vi "16TVTIMonitor.vi"() -> ()   [LabVIEW 2016]
uses:
  Utility/Monitor Communication/S16/VTI-cluster.ctl
  Utility/Monitor Communication/S16/VTI-control.ctl
  Instrument_Setup.vi
  Global/Global Variables/Data_Display_global.vi
panel:
  out "VTI":T1={"Temperatur (K)"=0.0, "Setpoint (K)"=0.0, "Rate (K/min)"=3.4572, "Heater (%)"=0.0, "NV (%)"=0.0, "Heater Manual"=FALSE, "NV Manual"=FALSE, "Go to Set"=FALSE, "Pressure"=0.0, "Heater SP"=0.0, "Valid?"=FALSE, "Set Heater SP"=FALSE, "Set NV SP"=FALSE, "Heater (%) Display"=3.4572, "NV (%) Display"=3.4572, "NV Setpoint"=0.0, "Change Heater Status"=FALSE, "Change NV Status"=FALSE, "Sample 3"=0.0, "Sample 2"=0.0, "Sweep-State"=FALSE, "Set Auto PID"=FALSE, "Auto PID"=FALSE, "Stopp"=FALSE, "Setpoint-Sweep"=0.0} {"NV (%) Display" format="%4_5f"; "Heater (%) Display" format="%4_5f"; "Pressure" format="%#4_5f"; "NV (%)" scale=0.0..100.0; "Heater (%)" scale=0.0..100.0; "Rate (K/min)" format="%#4_5f"; "Setpoint (K)" format="%6_5f"}
  in  "local error":errorcluster
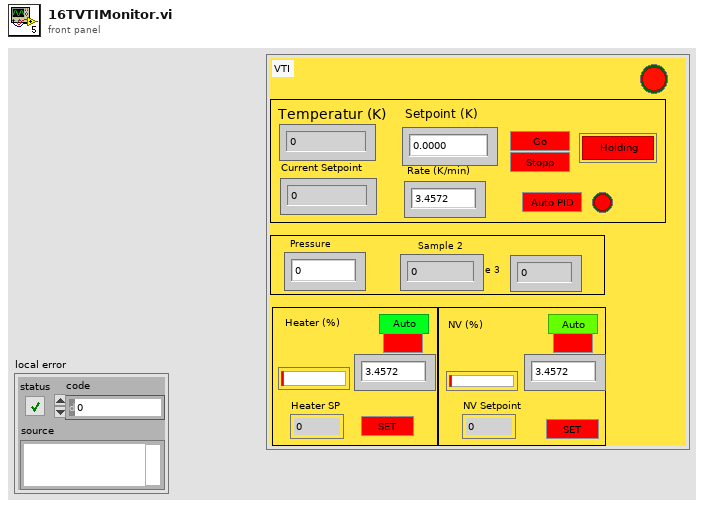
[diagram p1: front panel]
types:
  T1 = typedef "VTI-cluster.ctl" = cluster{"Temperatur (K)":dbl, "Setpoint (K)":dbl, "Rate (K/min)":dbl, "Heater (%)":dbl, "NV (%)":dbl, "Heater Manual":bool, "NV Manual":bool, "Go to Set":bool, "Pressure":dbl, "Heater SP":dbl, "Valid?":bool, "Set Heater SP":bool, "Set NV SP":bool, "Heater (%) Display":dbl, "NV (%) Display":dbl, "NV Setpoint":dbl, "Change Heater Status":bool, "Change NV Status":bool, "Sample 3":dbl, "Sample 2":dbl, "Sweep-State":bool, "Set Auto PID":bool, "Auto PID":bool, "Stopp":bool, "Setpoint-Sweep":dbl}
  T2 = typedef "VTI-control.ctl" = cluster{"Set VTI SP":bool, "Change NV Status":bool, "Set NV Setpoint":bool, "Change Heater Status":bool, "Set Heater Setpoint":bool, "Setpoint (K)":dbl, "Rate (K/min)":dbl, "Setpoint Heater":dbl, "Setpoint NV":dbl, "Change Auto PID":bool, "Stop Sweep":bool}
  T3 = typedef "ITCVersion.ctl" = enum16{"ITC502", "ITC503", "ITC601"}
  T4 = cluster{"Version":T3, "ControlTITC":i8, "ControlTCh":i8, "SampleTITC":i8, "SampleTCh":i8, "Instrument address":cluster{"Com Port":i32, "ISOBUS Address":i32, "GPIB Address":i16, "Communication":enum16{"RS232", "ISOBUS", "GPIB", "Gateway"}}}
  T5 = cluster{"Com Port":i32, "ISOBUS Address":i32, "GPIB Address":i16, "Communication":enum16{"RS232", "ISOBUS", "GPIB", "Gateway"}}
  T6 = enum32{"Bad", "Idle", "Run top level", "Running"}
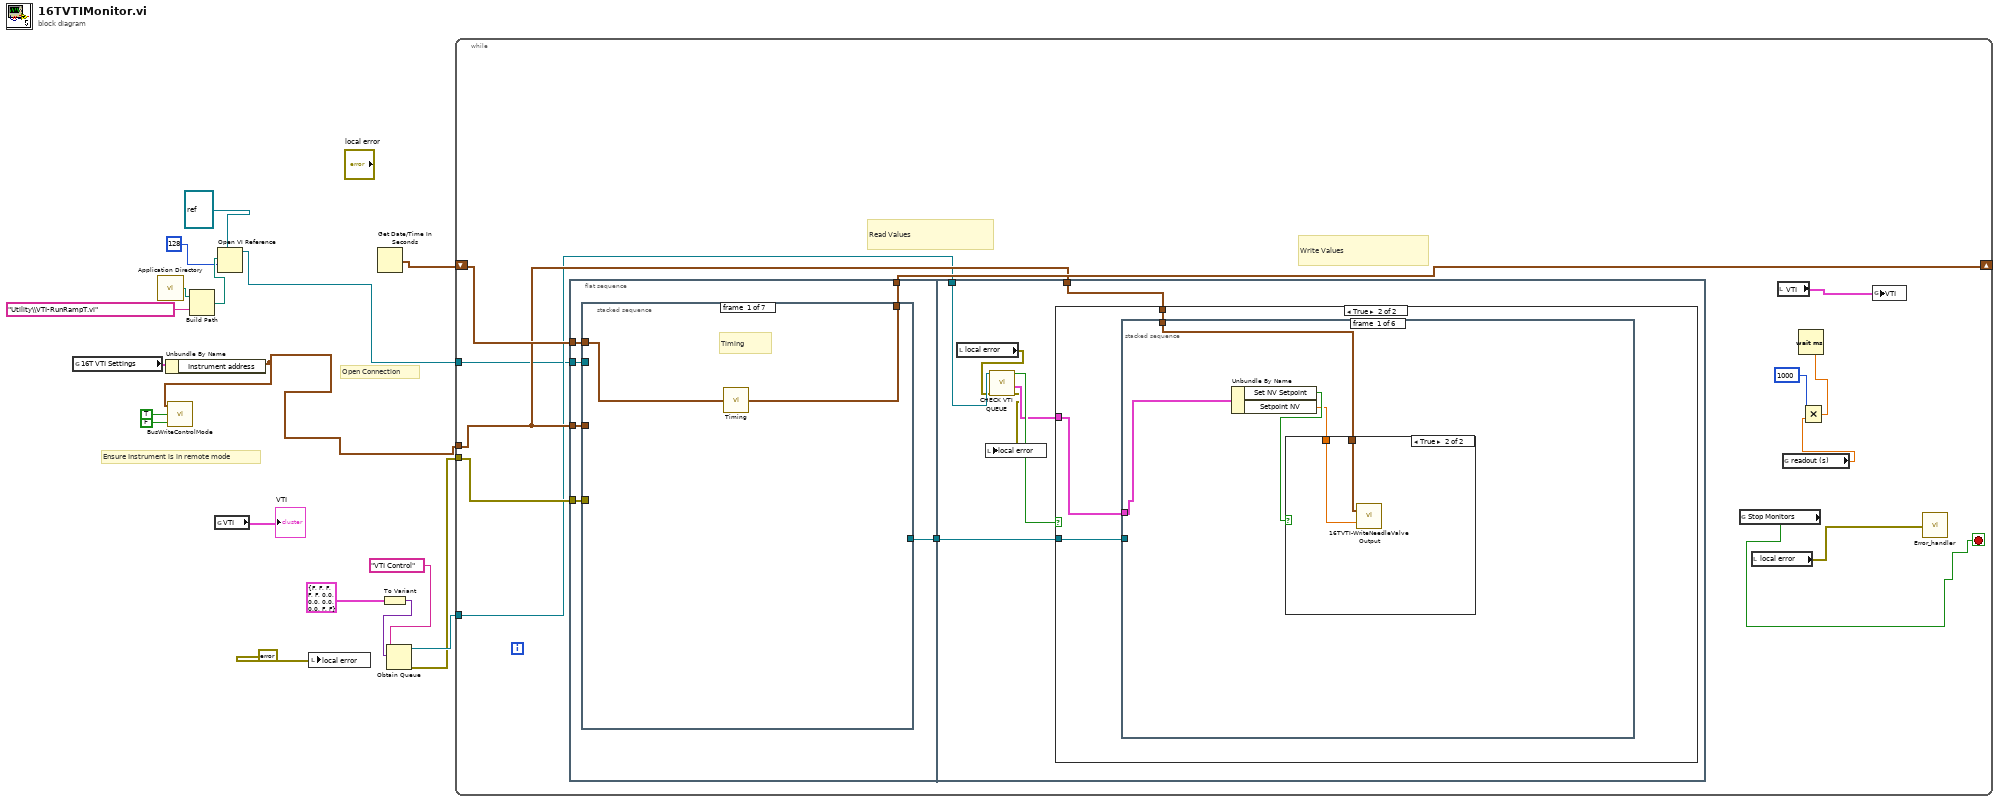
[diagram p0: block diagram]
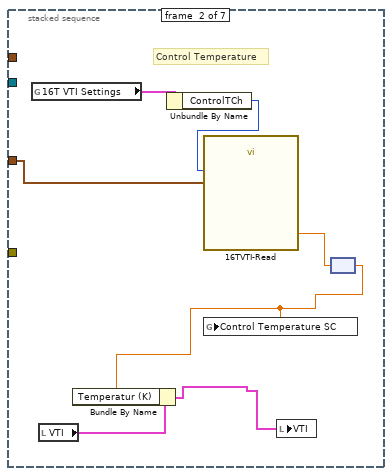
[diagram p2: hidden frame]
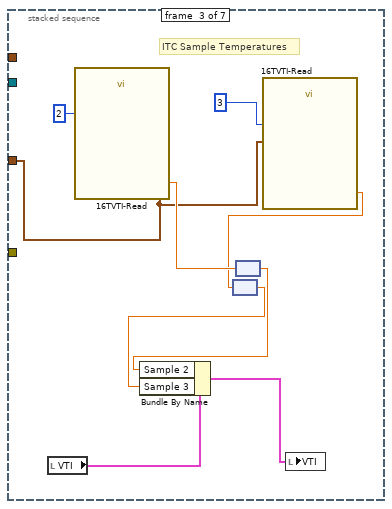
[diagram p3: hidden frame]
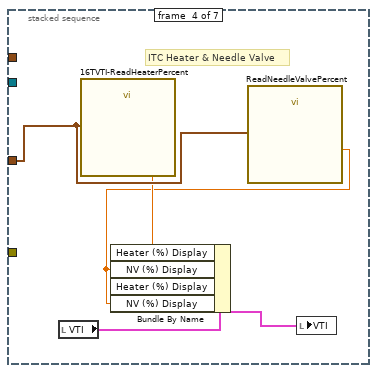
[diagram p4: hidden frame]
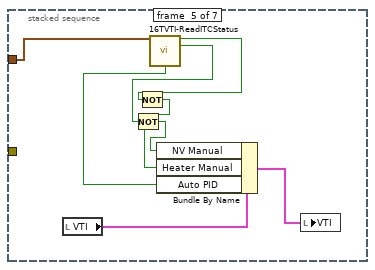
[diagram p5: hidden frame]
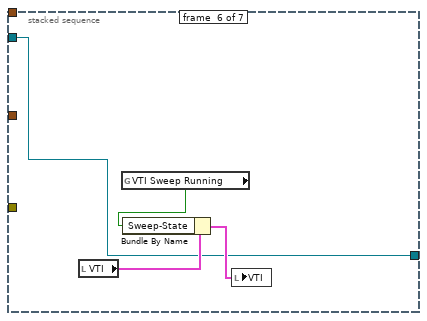
[diagram p6: hidden frame]
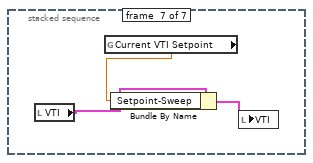
[diagram p7: hidden frame]
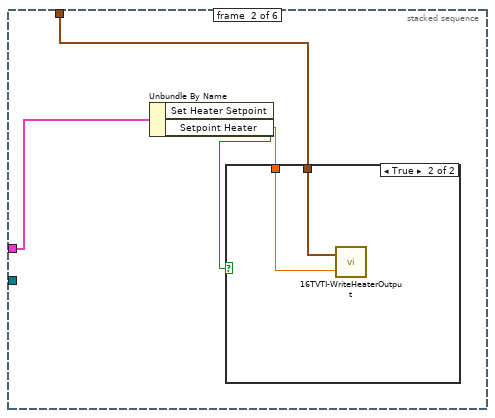
[diagram p10: hidden frame]
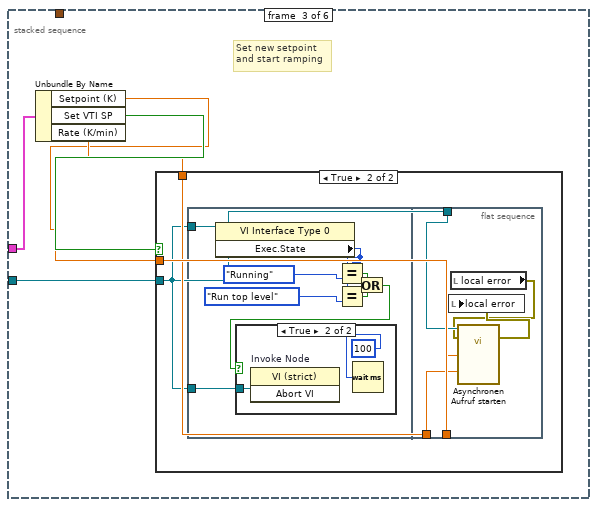
[diagram p12: hidden frame]
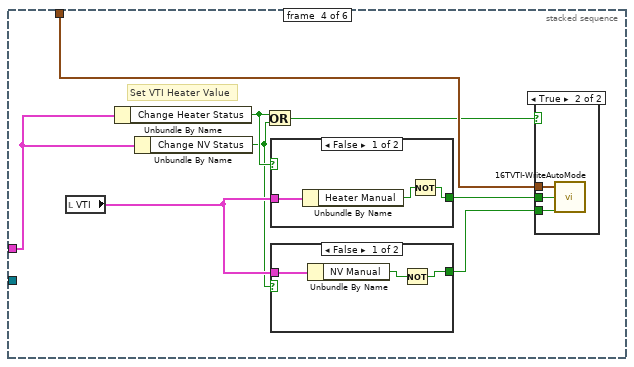
[diagram p15: hidden frame]
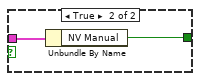
[diagram p17: hidden frame]
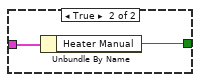
[diagram p18: hidden frame]
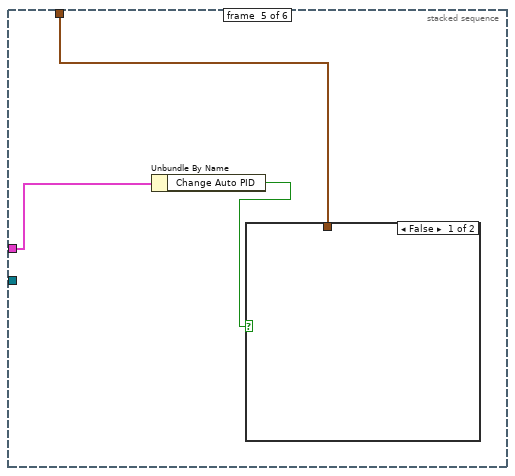
[diagram p19: hidden frame]
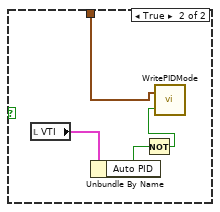
[diagram p20: hidden frame]
diagram:
  # "Ensure Instrument is in remote mode"
  # "Open Connection"
  n1 = global read "Instrument_Setup.vi" "16T VTI Settings"() -> (w4:T4)
  n2 = call <vilib>:"Application Directory.vi"() -> ("Application Directory"=w10:path)
  n3 = Unbundle By Name(w4) -> ("Instrument address"=w1:T5)
  n4 = call "BusWriteControlMode.vi"("Locked"=FALSE, "Remote"=TRUE, "Address"=w1) -> ()  [unwired: 1 out]
  n5 = Build Path(base path=w10, name or relative path="Utility\\VTI-RunRampT.vi") -> (appended path=w8:path)
  n6 = global read "Data_Display_global.vi" "VTI"() -> (→"VTI":T1)
  n7 = Open VI Reference(type specifier VI Refnum (for type only)=refnum<vi> refnum ("vi reference"), vi path=w8, options=128) -> (vi reference=w5:refnum<vi>)  [unwired: 3 in, 1 out]
  n8 = local write "local error"(errorcluster {"status"=FALSE, "code"=0, "source"=""} ("error constant")) -> ()
  n9 = Get Date/Time In Seconds() -> (seconds since 1Jan1904=w18:timestamp)
  n10 = To Variant(anything=T2 {"Set VTI SP"=FALSE, "Change NV Status"=FALSE, "Set NV Setpoint"=FALSE, "Change Heater Status"=FALSE, "Set Heater Setpoint"=FALSE, "Setpoint (K)"=0.0, "Rate (K/min)"=0.0, "Setpoint Heater"=0.0, "Setpoint NV"=0.0, "Change Auto PID"=FALSE, "Stop Sweep"=FALSE} ("VTI Control")) -> (Variant=w17:variant)
  n11 = Obtain Queue(name (unnamed)="VTI Control", element data type=w17) -> (queue out=w15:refnum<queue>, error out=w14:errorcluster)  [unwired: 3 in, 1 out]
  n12 = while {
    tunnel: w1 -> [w25]
    tunnel: w14 -> [w31]
    shift-right: [w26] -> _
    shift-left: w18 -> [w27]
    tunnel: w15 -> [w23]
    tunnel: w5 -> [w20]
    stop <- w21 stop-if-true
    # "Write Values"
    # "Read Values"
    n13 = flat-sequence {
      tunnel: w31 -> [w37]
      tunnel: w25 -> [w36]
      tunnel: w27 -> [w35]
      tunnel: [w34] -> w26
      tunnel: w20 -> [w33]
      tunnel: [w32] -> w19
      tunnel: w25 -> [w82]
      tunnel: w23 -> [w81]
      tunnel: w19 -> [w76]
      frame #0 {
        n14 = stacked-sequence {
          tunnel: w36 -> [_ w46 w50 w60 w64 _ _]
          tunnel: w37 -> [_ _ _ _ _ _ _]
          tunnel: w35 -> [w39 _ _ _ _ _ _]
          tunnel: [w38 _ _ _ _ _ _] -> w34
          tunnel: w33 -> [_ _ _ _ _ w70 _]
          tunnel: [_ _ _ _ _ w70 _] -> w32
          frame #0 {
            # "Timing"
            n15 = call "Timing.vi"("start time (s)"=w39) -> ("last reading (s)"=w38:timestamp)
          }
          frame #1 {
            # "Control Temperature"
            n16 = global read "Instrument_Setup.vi" "16T VTI Settings"() -> (w41:T4)
            n17 = local read "VTI"() -> (w45:T1)
            n18 = Unbundle By Name(w41) -> ("ControlTCh"=w40:i8)
            n19 = call "16TVTI-Read.vi"("Channel"=w40, "IO Info"=w46) -> ("Temperature"=w43:dbl[unit])  [unwired: 3 in, 2 out]
            n20 = node(w43) -> (w42:dbl)
            n21 = Bundle By Name(cluster=w45, "Temperatur (K)"=w42) -> (w44:T1)
            n22 = global write "Data_Display_global.vi" "Control Temperature SC"(w42) -> ()
            n23 = local write "VTI"(w44) -> ()
          }
          frame #2 {
            # "ITC Sample Temperatures"
            n24 = local read "VTI"() -> (w53:T1)
            n25 = call "16TVTI-Read.vi"("Channel"=i16 2, "IO Info"=w50) -> ("Temperature"=w54:dbl[unit])  [unwired: 3 in, 2 out]
            n26 = node(w54) -> (w48:dbl)
            n27 = call "16TVTI-Read.vi"("Channel"=i16 3, "IO Info"=w50) -> ("Temperature"=w49:dbl[unit])  [unwired: 3 in, 2 out]
            n28 = node(w49) -> (w47:dbl)
            n29 = Bundle By Name(cluster=w53, "Sample 2"=w48, "Sample 3"=w47) -> (w52:T1)
            n30 = local write "VTI"(w52) -> ()
          }
          frame #3 {
            # "ITC Heater & Needle Valve"
            n31 = local read "VTI"() -> (w58:T1)
            n32 = call "16TVTI-ReadHeaterPercent.vi"("ITC IO Info"=w60) -> ("Actual heater  %"=w57:dbl)  [unwired: 1 in, 1 out]
            n33 = call "ReadNeedleValvePercent.vi"("IO Info"=w60) -> ("Actual Needle Valve  %"=w56:dbl)  [unwired: 1 in, 1 out]
            n34 = Bundle By Name(cluster=w58, "Heater (%) Display"=w57, "NV (%) Display"=w56, "Heater (%) Display"=w57, "NV (%) Display"=w56) -> (w59:T1)
            n35 = local write "VTI"(w59) -> ()
          }
          frame #4 {
            n36 = local read "VTI"() -> (w68:T1)
            n37 = call "16TVTI-ReadITCStatus.vi"("ITC IO Info"=w64) -> ("Auto heat"=w66:bool, "Auto Needle Valve"=w65:bool, "Auto PID"=w61:bool)  [unwired: 4 in, 8 out]
            n38 = Not(x=w65) -> (.not. x?=w63:bool)
            n39 = Not(x=w66) -> (.not. x?=w62:bool)
            n40 = Bundle By Name(cluster=w68, "NV Manual"=w63, "Heater Manual"=w62, "Auto PID"=w61) -> (w67:T1)
            n41 = local write "VTI"(w67) -> ()
          }
          frame #5 {
            n42 = local read "VTI"() -> (w72:T1)
            n43 = global read "Data_Display_global.vi" "VTI Sweep Running"() -> (w69:bool)
            n44 = Bundle By Name(cluster=w72, "Sweep-State"=w69) -> (w71:T1)
            n45 = local write "VTI"(w71) -> ()
          }
          frame #6 {
            n46 = local read "VTI"() -> (w75:T1)
            n47 = global read "Data_Display_global.vi" "Current VTI Setpoint"() -> (w73:dbl)
            n48 = Bundle By Name(cluster=w75, "Setpoint-Sweep"=w73) -> (w74:T1)
            n49 = local write "VTI"(w74) -> ()
          }
        }
      }
      frame #1 {
        n50 = local read "local error"() -> (w78:errorcluster)
        n51 = call "CHECK VTI QUEUE.vi"("error in (no error)"=w78, "queue"=w81) -> ("error out"=w77:errorcluster, "VTI Control"=w79:T2, "New Entries?"=w80:bool)  [unwired: 6 in]
        n52 = local write "local error"(w77) -> ()
        n53 = case shown="True" w80 {
          tunnel: w82 -> [_ w85]
          tunnel: w79 -> [_ w84]
          tunnel: w76 -> [_ w83]
          frame False {
          }
          frame True {
            n54 = stacked-sequence {
              tunnel: w85 -> [w87 w92 _ w124 w143 _]
              tunnel: w84 -> [w89 w93 w102 w128 w142 w153]
              tunnel: w83 -> [_ _ w98 _ _ w152]
              frame #0 {
                n55 = Unbundle By Name(w89) -> ("Set NV Setpoint"=w88:bool, "Setpoint NV"=w86:dbl)
                n56 = case shown="True" w88 {
                  tunnel: w87 -> [_ w91]
                  tunnel: w86 -> [_ w90]
                  frame False {
                  }
                  frame True {
                    n57 = call "16TVTI-WriteNeedleValveOutput.vi"("Needle Valve Output (%"=w90, "ITC IO Info"=w91) -> ()  [unwired: 1 in, 1 out]
                  }
                }
              }
              frame #1 {
                n58 = Unbundle By Name(w93) -> ("Set Heater Setpoint"=w95:bool, "Setpoint Heater"=w94:dbl)
                n59 = case shown="True" w95 {
                  tunnel: w92 -> [_ w97]
                  tunnel: w94 -> [_ w96]
                  frame False {
                  }
                  frame True {
                    n60 = call "16TVTI-WriteHeaterOutput.vi"("Heater Output (%)"=w96, "ITC IO Info"=w97) -> ()  [unwired: 1 in, 1 out]
                  }
                }
              }
              frame #2 {
                # "Set new setpoint \nand start ramping"
                n61 = Unbundle By Name(w102) -> ("Setpoint (K)"=w99:dbl, "Set VTI SP"=w101:bool, "Rate (K/min)"=w100:dbl)
                n62 = case shown="True" w101 {
                  tunnel: w99 -> [_ w105]
                  tunnel: w100 -> [_ w104]
                  tunnel: w98 -> [_ w103]
                  frame False {
                  }
                  frame True {
                    n63 = flat-sequence {
                      tunnel: w103 -> [w113]
                      tunnel: w103 -> [w106]
                      tunnel: w105 -> [w120]
                      tunnel: w104 -> [w119]
                      tunnel: w103 -> [w118]
                      frame #0 {
                        n64 = property class="VI Interface Type 0"(reference=w113) -> ("Exec.State"=w107:T6)  [unwired: 1 in, 2 out]
                        n65 = Equal?(x=w107, y=T6."Running" ("LS 370 Monitor 2")) -> (x = y?=w111:bool)
                        n66 = Equal?(x=w107, y=T6."Run top level" ("LS 370 Monitor 2")) -> (x = y?=w112:bool)
                        n67 = Or(x=w111, y=w112) -> (x .or. y?=w110:bool)
                        n68 = case shown="True" w110 {
                          tunnel: w106 -> [_ w115]
                          frame False {
                          }
                          frame True {
                            n69 = invoke on="Invoke Node" class="VI (strict)" method="Abort VI"(reference=w115) -> ()  [unwired: 2 in, 3 out]
                            n70 = Wait (ms)(milliseconds to wait=100) -> ()  [unwired: 1 out]
                          }
                        }
                      }
                      frame #1 {
                        n71 = local read "local error"() -> (w116:errorcluster)
                        n72 = call-by-ref "Asynchronen Aufruf starten"(reference=w118, error in=w116, "Rate (K/min)"=w119, "Final T (K)"=w120) -> (error out=w117:errorcluster)  [unwired: 2 out]
                        n73 = local write "local error"(w117) -> ()
                      }
                    }
                  }
                }
              }
              frame #3 {
                # "Set VTI Heater Value"
                n74 = local read "VTI"() -> (w127:T1)
                n75 = Unbundle By Name(w128) -> ("Change Heater Status"=w123:bool)
                n76 = Unbundle By Name(w128) -> ("Change NV Status"=w121:bool)
                n77 = Or(x=w123, y=w121) -> (x .or. y?=w122:bool)
                n78 = case shown="False" w123 {
                  tunnel: w127 -> [w139 w141]
                  tunnel: [w137 w140] -> w125
                  frame False {
                    n79 = Unbundle By Name(w139) -> ("Heater Manual"=w138:bool)
                    n80 = Not(x=w138) -> (.not. x?=w137:bool)
                  }
                  frame True {
                    n81 = Unbundle By Name(w141) -> ("Heater Manual"=w140:bool)
                  }
                }
                n82 = case shown="False" w121 {
                  tunnel: w127 -> [w134 w136]
                  tunnel: [w132 w135] -> w126
                  frame False {
                    n83 = Unbundle By Name(w134) -> ("NV Manual"=w133:bool)
                    n84 = Not(x=w133) -> (.not. x?=w132:bool)
                  }
                  frame True {
                    n85 = Unbundle By Name(w136) -> ("NV Manual"=w135:bool)
                  }
                }
                n86 = case shown="True" w122 {
                  tunnel: w126 -> [_ w129]
                  tunnel: w125 -> [_ w130]
                  tunnel: w124 -> [_ w131]
                  frame False {
                  }
                  frame True {
                    n87 = call "16TVTI-WriteAutoMode.vi"("Auto Needle Valve"=w129, "Auto Heat"=w130, "Instrument address"=w131) -> ()  [unwired: 1 out]
                  }
                }
              }
              frame #4 {
                n88 = Unbundle By Name(w142) -> ("Change Auto PID"=w144:bool)
                n89 = case shown="False" w144 {
                  tunnel: w143 -> [_ w147]
                  frame False {
                  }
                  frame True {
                    n90 = local read "VTI"() -> (w148:T1)
                    n91 = Unbundle By Name(w148) -> ("Auto PID"=w146:bool)
                    n92 = Not(x=w146) -> (.not. x?=w145:bool)
                    n93 = call "WritePIDMode.vi"("Auto PID"=w145, "Instrument address"=w147) -> ()  [unwired: 1 in, 1 out]
                  }
                }
              }
              frame #5 {
                n94 = Unbundle By Name(w153) -> ("Stop Sweep"=w151:bool)
                n95 = global read "Data_Display_global.vi" "VTI Sweep Running"() -> (w149:bool)
                n96 = And(x=w151, y=w149) -> (x .and. y?=w150:bool)
                n97 = case shown="True" w150 {
                  tunnel: w152 -> [_ w154]
                  frame False {
                  }
                  frame True {
                    n98 = flat-sequence {
                      tunnel: w154 -> [w155]
                      frame #0 {
                        n99 = invoke on="Invoke Node" class="VI (strict)" method="Abort VI"(reference=w155) -> ()  [unwired: 2 in, 3 out]
                      }
                      frame #1 {
                        n100 = global write "Data_Display_global.vi" "VTI Sweep Running"(FALSE) -> ()
                      }
                    }
                  }
                }
              }
            }
          }
        }
      }
    }
    n101 = global read "Data_Display_global.vi" "Stop Monitors"() -> (w21:bool)
    n102 = local read "local error"() -> (w22:errorcluster)
    n103 = local read "VTI"() -> (w24:T1)
    n104 = global read "Instrument_Setup.vi" "readout (s)"() -> (w30:dbl)
    n105 = Multiply(x=1000, y=w30) -> (x*y=w29:dbl)
    n106 = Wait (ms)(milliseconds to wait=w29) -> ()  [unwired: 1 out]
    n107 = global write "Data_Display_global.vi" "VTI"(w24) -> ()
    n108 = call "Error_handler.vi"("error constant"=w22) -> ()
  }
